vi "poly test (bool).vi"(1 "Boolean":bool) -> (0 "Boolean out":bool)   [LabVIEW 2012]
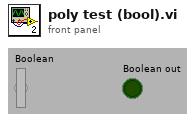
[diagram p1: front panel]
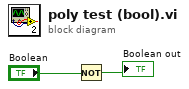
[diagram p0: block diagram]
diagram:
  n1 = Not(x="Boolean") -> (.not. x?=→"Boolean out":bool)
